vi "ClearFaults.vi"(11 "class data in":refnum<class "AnalogComparator.lvclass">) -> (3 "class data out":refnum<class "AnalogComparator.lvclass">)   [LabVIEW 2019, in "AnalogComparator.lvclass"]
uses:
  AnalogComparator.lvclass
  AnalogComparator.lvclass/AnalogComparator.ctl
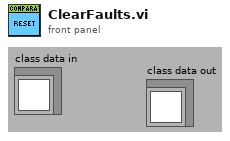
[diagram p1: front panel]
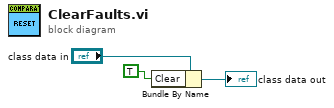
[diagram p0: block diagram]
diagram:
  n1 = Bundle By Name(cluster="class data in", "Clear"=TRUE ("Status")) -> (→"class data out":refnum<class "AnalogComparator.lvclass">)
